vi "uA_daq_Initial_Aquire_mode.vi"(8 "error in":errorcluster, 9 "ADC_Ch":string="/ai3", 10 "Acquire Mode":enum16{"Streaming", "Read All", "Stop"}(ring), 11 "USB DAQ":tag) -> (0 "error out":errorcluster, 3 "Refnum out":refnum<k21>)   [LabVIEW 2015]
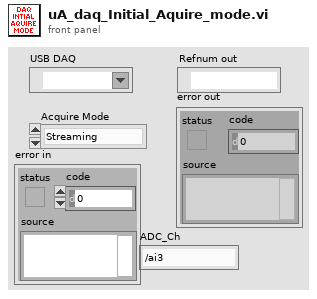
[diagram p1: front panel]
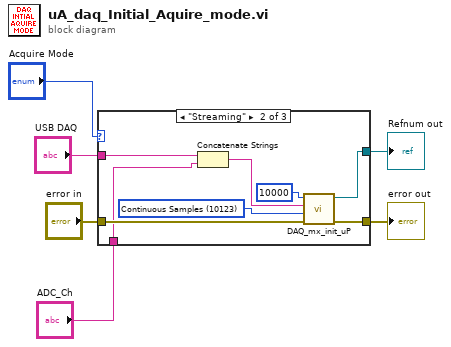
[diagram p0: block diagram]
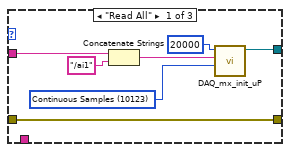
[diagram p2: hidden frame]
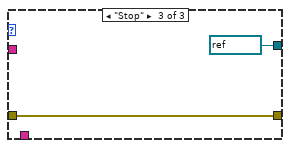
[diagram p3: hidden frame]
diagram:
  n1 = case shown="\"Streaming\"" "Acquire Mode" {
    tunnel: [w9 w18 refnum<k21> "Stop" ("task out")] -> w5
    tunnel: "USB DAQ" -> [w8 w17 _]
    tunnel: "error in" -> [w7 w16 w22]
    tunnel: [w7 w15 w22] -> w2
    tunnel: "ADC_Ch" -> [_ w14 _]
    frame "Read All" {
      w11 = 10123 items=["Finite Samples"=10178, "Continuous Samples"=10123, "Hardware Timed Single Point"=12522] ("sample mode")
      n2 = Concatenate Strings(w8, "/ai1" ("string")) -> (w12:string)
      n3 = call "DAQ_mx_init_uP.vi"("sample mode"=w11, "physical channel"=w12, "number of samples"=20000 ("samples")) -> ("task out"=w9:refnum<k21>)  [unwired: 7 in, 1 out]
    }
    frame "Streaming" {
      w19 = 10123 items=["Finite Samples"=10178, "Continuous Samples"=10123, "Hardware Timed Single Point"=12522] ("sample mode")
      n4 = Concatenate Strings(w17, w14) -> (w20:string)
      n5 = call "DAQ_mx_init_uP.vi"("error in"=w16, "sample mode"=w19, "physical channel"=w20, "number of samples"=10000 ("samples")) -> ("error out"=w15:errorcluster, "task out"=w18:refnum<k21>)  [unwired: 6 in]
    }
    frame "Stop" {
    }
  }
  "Refnum out" <- w5
  "error out" <- w2
